vi "SR830_Setup.vi"(2 "SR830 Settings Cluster":T1={"VISA"="GPIB0::17::INSTR", "Display Channel 2"={" display"=0, " ratio"=0, "output"=1}, "Display Channel 1"={" display"=0, " ratio"=0, "output"=1}, "Time constant"={"time constant\n(10 µs : 0) "=12, "slope (6 dB/oct)"=3}, "Sensitivity"={"sensitivity\n2nV/fA"=0, "dyn reserve\n(low noise:2)"=2, "ref. phase"=0.0, "automeasure"=FALSE}, "Offset - Expand."={"Expand (0: x1)"=0, "Offset/Expand Parameter (1: X)"=0, "Manual Offset (0)"=0.0}, "Reference"={"ref. source"=TRUE, "osc.harm# "=1, "osc. freq"=22.08, "osc. ampl."=5.0, "ref. trigger"=0}, "Lock In 1 sync"={"sync filter"=FALSE, "line filter\n(off:0)"=0}, "Lock In 1 input"={"input"=1, "ground"=FALSE, "couple"=TRUE}} {"Lock In 1 input"."input" items=["A", "A-B", "I (1 M gain)", "I (100 M gain)"]; "Lock In 1 sync"."line filter\n(off:0)" items=["OFF", "line", "2 x line", "both"]; "Reference"."ref. trigger" items=["sine", "pos edge", "neg edge"]; "Reference"."osc.harm#" min=1 max=19999; "Reference"."osc. ampl." format="%.3f"; "Reference"."osc. freq" format="%.3f"; "Offset - Expand."."Offset/Expand Parameter (1: X)" items=["X"=1, "Y"=2, "R"=3]; "Offset - Expand."."Expand (0: x1)" items=["X", "Y", "R"]; "Sensitivity"."sensitivity\n2nV/fA" items=["2 nV/fA", "5 nV/fA", "10 nV/fA", "20 nV/fA", "50 nV/fA", "100 nV/fA", "200 nV/fA", "500 nV/fA", "1 µV /pA", "2 µV/pA", "5 µV/pA", "10 µV/pA", "20 µV/pA", "50 µV/pA", "100 µV/pA", "200 µV/pA", "500 µV/pA", "1 mV/nA", "2 mV/nA", "5 mV/nA", "10 mV/nA", "20 mV/nA", "50 mV/nA", "100 mV/nA", "200 mV/nA", "500 mV/nA", "1 V/µA"]; "Sensitivity"."dyn reserve\n(low noise:2)" scale=0.0..2.0 scale format="%.2f"; "Sensitivity"."ref. phase" format="%.2f"; "Time constant"."slope (6 dB/oct)" items=["6 dB/oct", "12 dB/oct", "18 dB/oct", "24 dB/oct"]; "Time constant"."time constant\n(10 µs : 0)" items=["10 µs", "30 µs", "100 µs", "300 µs", "1 ms", "3 ms", "10 ms", "30 ms", "100 ms", "300 ms", "1 s", "3 s", "10 s", "30 s", "100 s", "300 s", "1 ks", "3 ks", "10 ks", "30 ks"]; "Display Channel 1"."output" items=["display", "X"]; "Display Channel 1"."ratio" items=["none", "aux in 1", "aux in 2"]; "Display Channel 1"."display" items=["X", "R", "X Noise", "Aux In 1", "Aux In 2"]; "Display Channel 2"."output" items=["display", "Y"]; "Display Channel 2"."ratio" items=["none", "aux in 3", "aux in 4"]; "Display Channel 2"."display" items=["Y", "@", "Y Noise", "Aux In 3", "Aux In 4"]}) -> ()   [LabVIEW 2019]
uses:
  Monitor Communication/SR830/SR830-Settings-Cluster.ctl
  Equipment/Stanford Research 830/Stanford Research 830.lvlib
panel:
  # "float\nground"
  # "AC\nDC"
  # "on\noff"
  # "int\next"
  # "on\noff"
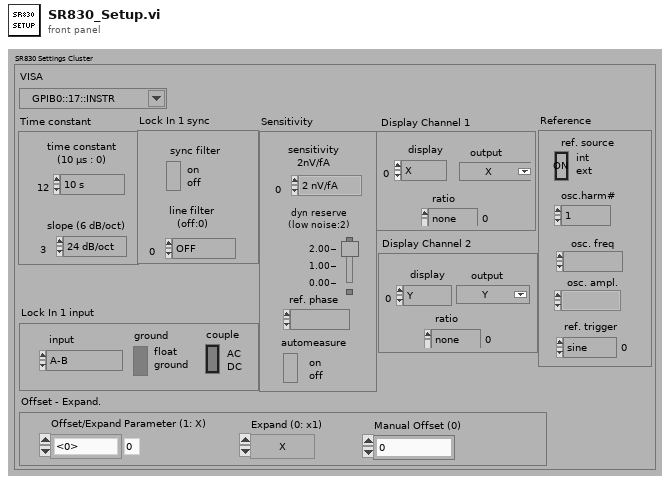
[diagram p1: front panel]
types:
  T1 = typedef "SR830-Settings-Cluster.ctl" = cluster{"VISA":refnum<visa-resource-name>, "Display Channel 2":cluster{" display":i32, " ratio":u16, "output":u16}, "Display Channel 1":cluster{" display":i32, " ratio":u16, "output":u16}, "Time constant":cluster{"time constant\n(10 µs : 0) ":i32, "slope (6 dB/oct)":i32}, "Sensitivity":cluster{"sensitivity\n2nV/fA":i32, "dyn reserve\n(low noise:2)":i16, "ref. phase":ext, "automeasure":bool}, "Offset - Expand.":cluster{"Expand (0: x1)":u16, "Offset/Expand Parameter (1: X)":u16, "Manual Offset (0)":dbl}, "Reference":cluster{"ref. source":bool, "osc.harm# ":u16, "osc. freq":ext, "osc. ampl.":ext, "ref. trigger":u16}, "Lock In 1 sync":cluster{"sync filter":bool, "line filter\n(off:0)":i32}, "Lock In 1 input":cluster{"input":u16, "ground":bool, "couple":bool}}
  T2 = cluster{" display":i32, " ratio":u16, "output":u16}
  T3 = cluster{"time constant\n(10 µs : 0) ":i32, "slope (6 dB/oct)":i32}
  T4 = cluster{"sensitivity\n2nV/fA":i32, "dyn reserve\n(low noise:2)":i16, "ref. phase":ext, "automeasure":bool}
  T5 = cluster{"Expand (0: x1)":u16, "Offset/Expand Parameter (1: X)":u16, "Manual Offset (0)":dbl}
  T6 = cluster{"ref. source":bool, "osc.harm# ":u16, "osc. freq":ext, "osc. ampl.":ext, "ref. trigger":u16}
  T7 = cluster{"sync filter":bool, "line filter\n(off:0)":i32}
  T8 = cluster{"input":u16, "ground":bool, "couple":bool}
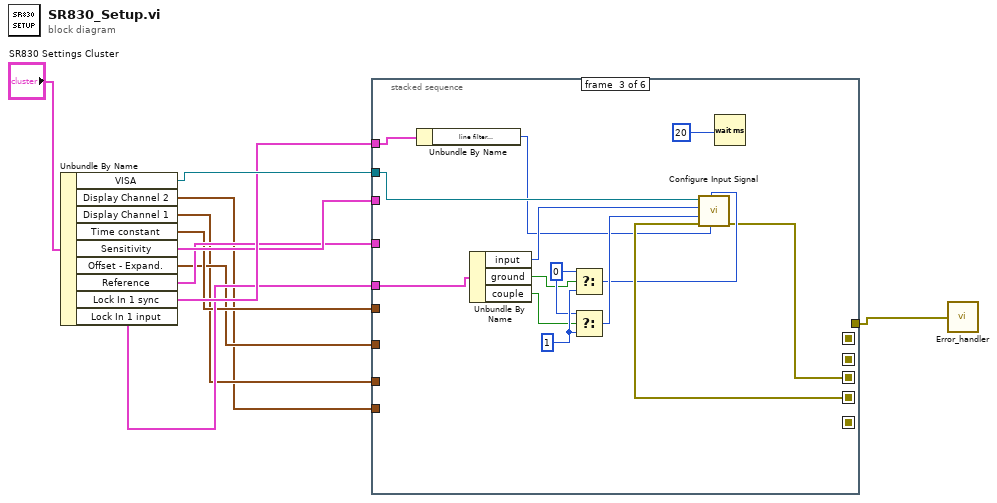
[diagram p0: block diagram]
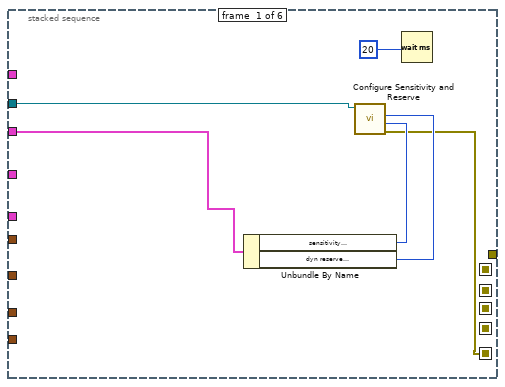
[diagram p2: hidden frame]
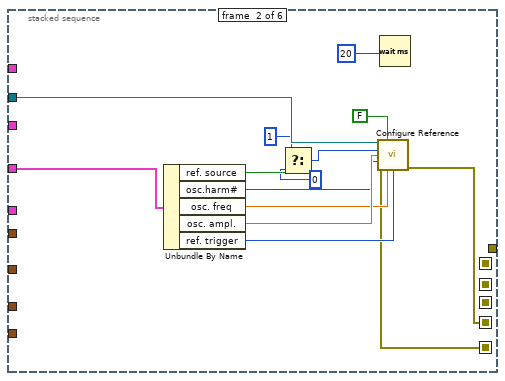
[diagram p3: hidden frame]
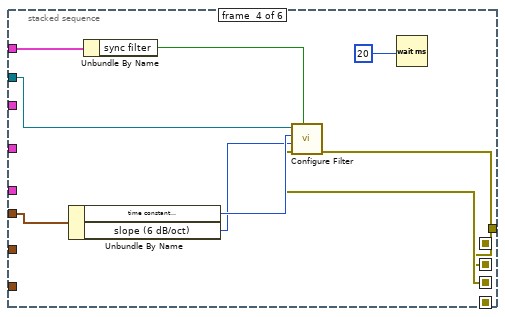
[diagram p4: hidden frame]
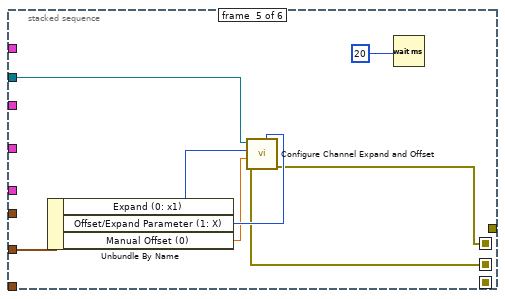
[diagram p5: hidden frame]
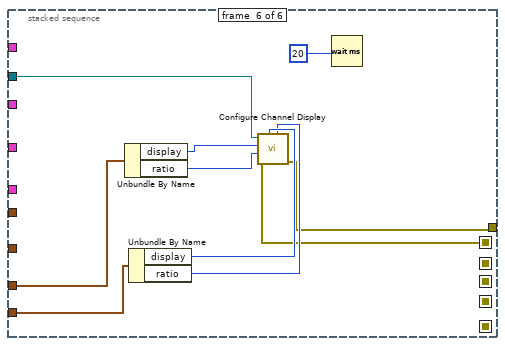
[diagram p6: hidden frame]
diagram:
  n1 = Unbundle By Name("SR830 Settings Cluster") -> ("VISA"=w11:refnum<visa-resource-name>, "Display Channel 2"=w3:T2, "Display Channel 1"=w4:T2, "Time constant"=w6:T3, "Sensitivity"=w9:T4, "Offset - Expand."=w5:T5, "Reference"=w8:T6, "Lock In 1 sync"=w10:T7, "Lock In 1 input"=w7:T8)
  n2 = stacked-sequence {
    seq-local: [w14 _ _ _ _ _] -> [_ w22 _ _ _ _]
    seq-local: [_ w21 _ _ _ _] -> [_ _ w44 _ _ _]
    seq-local: [_ _ w35 _ _ _] -> [_ _ _ w50 _ _]
    seq-local: [_ _ _ w49 _ _] -> [_ _ _ _ w57 _]
    seq-local: [_ _ _ _ w56 _] -> [_ _ _ _ _ w65]
    tunnel: w11 -> [w15 w31 w45 w53 w58 w66]
    tunnel: w7 -> [_ _ w43 _ _ _]
    tunnel: w8 -> [_ w20 _ _ _ _]
    tunnel: w9 -> [w13 _ _ _ _ _]
    tunnel: w6 -> [_ _ _ w54 _ _]
    tunnel: w5 -> [_ _ _ _ w62 _]
    tunnel: w4 -> [_ _ _ _ _ w72]
    tunnel: w3 -> [_ _ _ _ _ w71]
    tunnel: w10 -> [_ _ w34 w48 _ _]
    tunnel: [_ _ _ _ _ w64] -> w2
    frame #0 {
      n3 = Unbundle By Name(w13) -> ("sensitivity\n2nV/fA"=w17:i32, "dyn reserve\n(low noise:2)"=w16:i16)
      n4 = call "Configure Sensitivity and Reserve.vi"("Sensitivity (-1: Auto gain)"=w17, "Dynamic Reserve (-1: Auto Reserve)"=w16, "VISA resource name"=w15) -> ("error out"=w14:errorcluster)  [unwired: 7 in, 1 out]
      n5 = Wait (ms)(milliseconds to wait=20) -> ()  [unwired: 1 out]
    }
    frame #1 {
      n6 = Unbundle By Name(w20) -> ("ref. source"=w30:bool, "osc.harm#"=w25:u16, "osc. freq"=w24:ext, "osc. ampl."=w26:ext, "ref. trigger"=w23:u16)
      n7 = Select(t=1, s=w30, f=0) -> (s? t:f=w29:i32)
      n8 = call "Configure Reference.vi"("VISA resource name"=w31, "Auto Phase (T: Enabled)"=FALSE, "Reference Source (1: Internal)"=w29, "Sine Output Amplitude (1 V)"=w26, "Detection Harmonic Number (1)"=w25, "error in (no error)"=w22, "Internal Reference Frequency (1000 Hz)"=w24, "External Reference Trigger (0: Sine Zero Crossing)"=w23) -> ("error out"=w21:errorcluster)  [unwired: 6 in, 1 out]
      n9 = Wait (ms)(milliseconds to wait=20) -> ()  [unwired: 1 out]
    }
    frame #2 {
      w41 = 1
      w40 = 0
      n10 = Unbundle By Name(w34) -> ("line filter\n(off:0)"=w33:i32)
      n11 = Unbundle By Name(w43) -> ("input"=w42:u16, "ground"=w37:bool, "couple"=w36:bool)
      n12 = Select(t=w40, s=w37, f=w41) -> (s? t:f=w38:i32)
      n13 = Select(t=w40, s=w36, f=w41) -> (s? t:f=w39:i32)
      n14 = call "Configure Input Signal.vi"("Input Notch Filter (0: None)"=w33, "Input Shield Grounding (0: Float)"=w38, "error in (no error)"=w44, "Input Coupling (0: AC)"=w39, "Input Connection (0: Single-Ended Voltage)"=w42, "VISA resource name"=w45) -> ("error out"=w35:errorcluster)  [unwired: 4 in, 1 out]
      n15 = Wait (ms)(milliseconds to wait=20) -> ()  [unwired: 1 out]
    }
    frame #3 {
      n16 = Unbundle By Name(w54) -> ("time constant\n(10 µs : 0)"=w52:i32, "slope (6 dB/oct)"=w51:i32)
      n17 = Unbundle By Name(w48) -> ("sync filter"=w47:bool)
      n18 = call "Configure Filter.vi"("Enable Sync Filter (F: Disable)"=w47, "error in (no error)"=w50, "Low Pass Filter Slope (1: 12dB/oct)"=w51, "Time Constant (8: 100ms)"=w52, "VISA resource name"=w53) -> ("error out"=w49:errorcluster)  [unwired: 5 in, 1 out]
      n19 = Wait (ms)(milliseconds to wait=20) -> ()  [unwired: 1 out]
    }
    frame #4 {
      n20 = Unbundle By Name(w62) -> ("Expand (0: x1)"=w61:u16, "Offset/Expand Parameter (1: X)"=w60:u16, "Manual Offset (0)"=w59:dbl)
      n21 = call "Configure Channel Expand and Offset.vi"("Manual Offset (0)"=w60, "error in (no error)"=w57, "Expand (0: x1)"=w59, "Offset/Expand Parameter (1: X)"=w61, "VISA resource name"=w58) -> ("error out"=w56:errorcluster)  [unwired: 5 in, 1 out]
      n22 = Wait (ms)(milliseconds to wait=20) -> ()  [unwired: 1 out]
    }
    frame #5 {
      n23 = Unbundle By Name(w72) -> ("display"=w70:i32, "ratio"=w69:u16)
      n24 = Unbundle By Name(w71) -> ("display"=w68:i32, "ratio"=w67:u16)
      n25 = call "Configure Channel Display.vi"("Channel 2 Display With Ratio (0: None)"=w67, "Channel 2 Display  (0: Y)"=w68, "error in (no error)"=w65, "Channel 1 Display With Ratio (0: None)"=w69, "Channel 1 Display (0: X)"=w70, "VISA resource name"=w66) -> ("error out"=w64:errorcluster)  [unwired: 4 in, 1 out]
      n26 = Wait (ms)(milliseconds to wait=20) -> ()  [unwired: 1 out]
    }
  }
  n27 = call "Error_handler.vi"("error constant"=w2) -> ()
